vi "fontmontant detector.vi"() -> ()   [LabVIEW 2019]
uses:
  <vilib>/rvi/Emulation/niFpgaGetClockAttributes.vi
  <vilib>/rvi/Emulation/niFpgaSctlEmulationGetInTimedLoop.vi
  <vilib>/rvi/Emulation/niFpgaEmulationReportErrorSimple.vi
  <vilib>/rvi/eio/common/nirviEmuTemplateMethod_errors.vi
  <vilib>/rvi/Emulation/niFpgaCriticalErrorInLSC.vi
  <vilib>/eio/EIONode/EIONode.xnode
panel:
  in  "stop":bool
  in  "Reset":bool
  out "RisingEdge Counter":i16
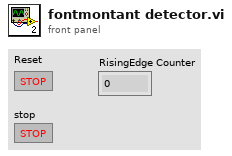
[diagram p1: front panel]
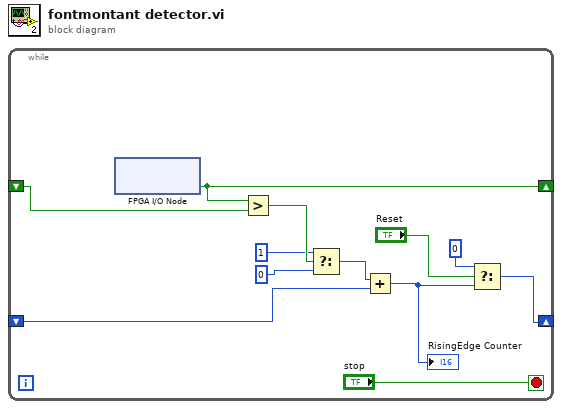
[diagram p0: block diagram]
diagram:
  n1 = while {
    shift-right: [w12] -> _
    shift-left: _ -> [w11]
    shift-right: [w2] -> _
    shift-left: _ -> [w7]
    stop <- "stop" stop-if-true
    n2 = xnode "FPGA I/O Node"() -> ("Button0"=w12:bool)  [unwired: 1 in, 1 out]
    n3 = Greater?(x=w12, y=w11) -> (0:w10:bool)
    n4 = Select(t=i16 1, s=w10, f=i16 0) -> (s? t:f=w6:i16)
    n5 = Add(x=w6, y=w7) -> (x+y=w4:i16)
    "RisingEdge Counter" <- w4
    n6 = Select(t=i16 0, s="Reset", f=w4) -> (s? t:f=w2:i16)
  }
